vi "DriveControl.vi"(5 "RobotDriveDevRef":T1={"DevStatus"={"status"=FALSE, "code"=0, "source"=""}, "Motors[]"=[], "Square Inputs"=FALSE, "Max Output"=1.0, "Isochronous"=FALSE}, 7 "Xvalue of Target":dbl, 8 "Right axis value":dbl, 9 "Left axis value":dbl, 10 "Lower Bound":dbl, 11 "Upper Bound":dbl) -> ()   [LabVIEW 2011]
uses:
  <vilib>/Rock Robotics/WPI/RobotDrive/WPI_RobotDriveDevRef.ctl
  <vilib>/Rock Robotics/WPI/MotorControl/WPI_MotorControlDeviceRef.ctl
  <vilib>/Rock Robotics/SystemInterfaces/Typedef/FPGA_TypedefDigitalModule.ctl
  <vilib>/Rock Robotics/SystemInterfaces/DIO/FPGA_DIOPWMChannel.ctl
  <vilib>/Rock Robotics/WPI/PWM/WPI_PWMDeadband.ctl
  <vilib>/Rock Robotics/WPI/CAN/Jaguar/SubVIs/WPI_CANJaguar_ControlMode.ctl
  <vilib>/Rock Robotics/WPI/PWM/WPI_PWMTransform_ConPane.ctl
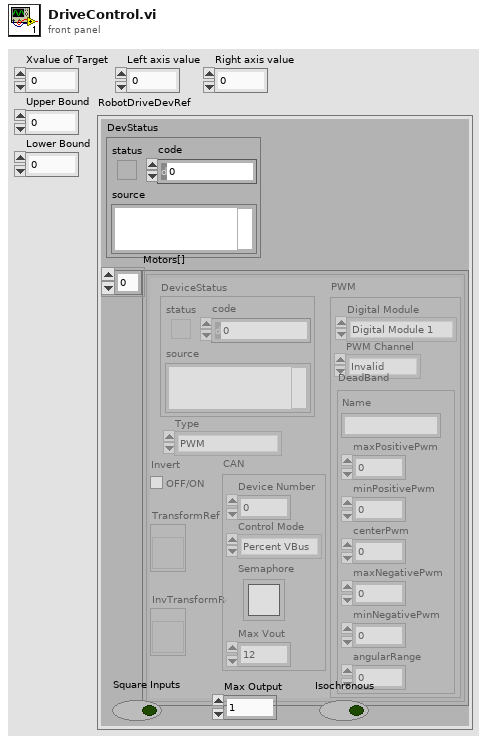
[diagram p1: front panel]
types:
  T1 = typedef "WPI_RobotDriveDevRef.ctl" = cluster{"DevStatus":errorcluster, "Motors[]":T2[], "Square Inputs":bool, "Max Output":dbl, "Isochronous":bool}
  T2 = typedef "WPI_MotorControlDeviceRef.ctl" = cluster{"DeviceStatus":errorcluster, "Type":enum16{"PWM", "CAN"}, "PWM":cluster{"Digital Module":T3, "PWM Channel":T4, "DeadBand":T5}, "CAN":cluster{"Device Number":u8, "Control Mode":T6, "Semaphore":T7, "Max Vout":dbl}, "Invert":bool, "TransformRef":T8, "InvTransformRef":T8}
  T3 = typedef "FPGA_TypedefDigitalModule.ctl" = enum16{"Digital Module 1", "Digital Module 2"}
  T4 = typedef "FPGA_DIOPWMChannel.ctl" = enum8{"PWM 1", "PWM 2", "PWM 3", "PWM 4", "PWM 5", "PWM 6", "PWM 7", "PWM 8", "PWM 9", "PWM 10", "Invalid"}
  T5 = typedef "WPI_PWMDeadband.ctl" = cluster{"Name":string, "maxPositivePwm":i32, "minPositivePwm":i32, "centerPwm":i32, "maxNegativePwm":i32, "minNegativePwm":i32, "angularRange":u16}
  T6 = typedef "WPI_CANJaguar_ControlMode.ctl" = enum8{"Percent VBus", "Current", "Speed", "Position", "Voltage"}
  T7 = typedef "Semaphore RefNum" = refnum<k1>
  T8 = typedef "WPI_PWMTransform_ConPane.ctl" = refnum<vi>
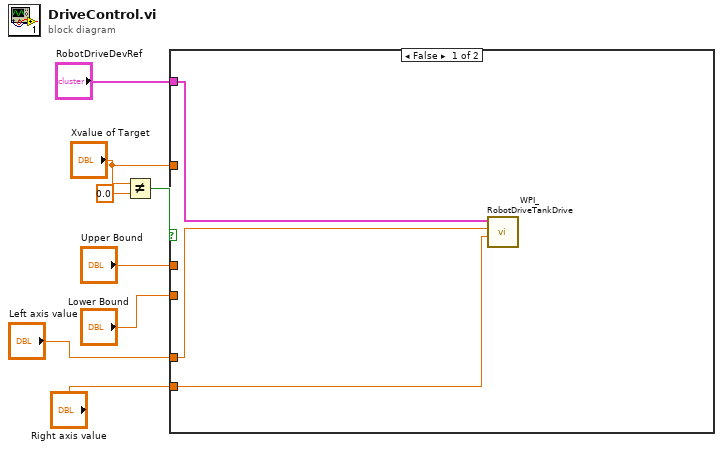
[diagram p0: block diagram]
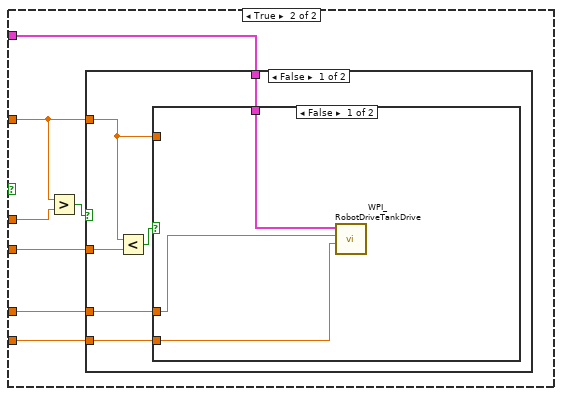
[diagram p2: hidden frame]
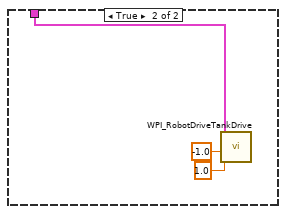
[diagram p3: hidden frame]
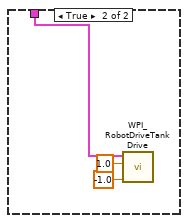
[diagram p4: hidden frame]
diagram:
  n1 = Not Equal?(x="Xvalue of Target", y=0.0) -> (x != y?=w7:bool)
  n2 = case shown="False" w7 {
    tunnel: "Xvalue of Target" -> [_ w16]
    tunnel: "Upper Bound" -> [_ w18]
    tunnel: "Lower Bound" -> [_ w15]
    tunnel: "RobotDriveDevRef" -> [w11 w14]
    tunnel: "Left axis value" -> [w9 w13]
    tunnel: "Right axis value" -> [w10 w12]
    frame False {
      n3 = call <vilib>:"WPI_RobotDriveTankDrive.vi"("Right axis value"=w10, "Left axis value"=w9, "RobotDriveDevRef"=w11) -> ()  [unwired: 7 in, 2 out]
    }
    frame True {
      n4 = Greater?(x=w16, y=w18) -> (0:w17:bool)
      n5 = case shown="False" w17 {
        tunnel: w16 -> [w19 _]
        tunnel: w15 -> [w23 _]
        tunnel: w14 -> [w22 w33]
        tunnel: w13 -> [w21 _]
        tunnel: w12 -> [w20 _]
        frame False {
          n6 = Less?(x=w19, y=w23) -> (x < y?=w24:bool)
          n7 = case shown="False" w24 {
            tunnel: w22 -> [w27 w30]
            tunnel: w21 -> [w26 _]
            tunnel: w20 -> [w25 _]
            tunnel: w19 -> [_ _]
            frame False {
              n8 = call <vilib>:"WPI_RobotDriveTankDrive.vi"("Right axis value"=w25, "Left axis value"=w26, "RobotDriveDevRef"=w27) -> ()  [unwired: 7 in, 2 out]
            }
            frame True {
              n9 = call <vilib>:"WPI_RobotDriveTankDrive.vi"("Right axis value"=-1.0, "Left axis value"=1.0, "RobotDriveDevRef"=w30) -> ()  [unwired: 7 in, 2 out]
            }
          }
        }
        frame True {
          n10 = call <vilib>:"WPI_RobotDriveTankDrive.vi"("Right axis value"=-1.0, "Left axis value"=1.0, "RobotDriveDevRef"=w33) -> ()  [unwired: 7 in, 2 out]
        }
      }
    }
  }
